vi "Position Arm.vi"(11 "Enum":enum16{"Start", "Run"}(ring)) -> (3 "Finished?":bool)   [LabVIEW 2012]
panel:
  in  "y":dbl=2.0
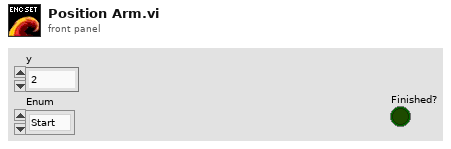
[diagram p1: front panel]
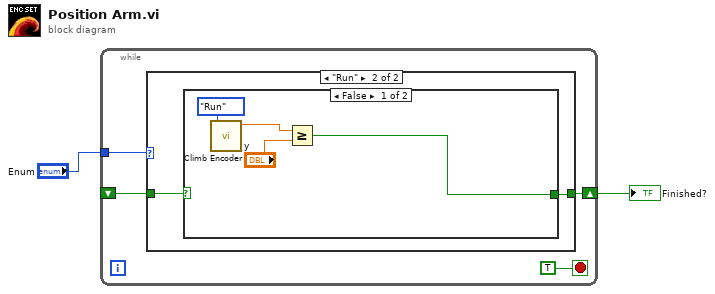
[diagram p0: block diagram]
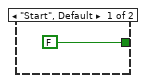
[diagram p2: hidden frame]
diagram:
  n1 = while {
    tunnel: "Enum" -> [w5]
    shift-right: [w4] -> w1
    shift-left: _ -> [w3]
    stop <- TRUE stop-if-true
    n2 = case shown="\"Run\"" w5 {
      tunnel: [FALSE w9] -> w4
      tunnel: w3 -> [_ w8]
      frame "Start", Default {
      }
      frame "Run" {
        n3 = case shown="False" w8 {
          selector: w8 -> [_ w14]
          tunnel: [w10 w14] -> w9
          frame False {
            n4 = call "Climb Encoder.vi"("Enum"=enum16{"Start", "Run", "End"}."Run") -> ("Distance"=w12:dbl)  [unwired: 10 in]
            n5 = Greater Or Equal?(x=w12, y="y") -> (x >= y?=w10:bool)
          }
          frame True {
          }
        }
      }
    }
  }
  "Finished?" <- w1
